vi "Auto-Calibrate.vi"(6 "Uncertainty (%) Vin":dbl=1.0, 7 "Uncertainty (%) Vout":dbl=1.0, 10 "V_in (V)":dbl=5.0) -> (0 "Uncertainty Calib Temp":dbl=1.0, 1 "Calib Temperature":dbl=292.15, 2 "Uncertainty (%) Thermistor":dbl=2.872472092283147, 3 "Calibration Resistance (ohms)":dbl=7684.457551235735)   [LabVIEW 2012]
panel:
  in  "Uncertainty (%) Resistor":dbl=1.0
  in  "Resistor (ohms)":dbl=10000.0
  in  "Uncertainty (%) Temp":dbl=1.0
  in  "Temperature (K)":dbl=292.15
  # "Options"
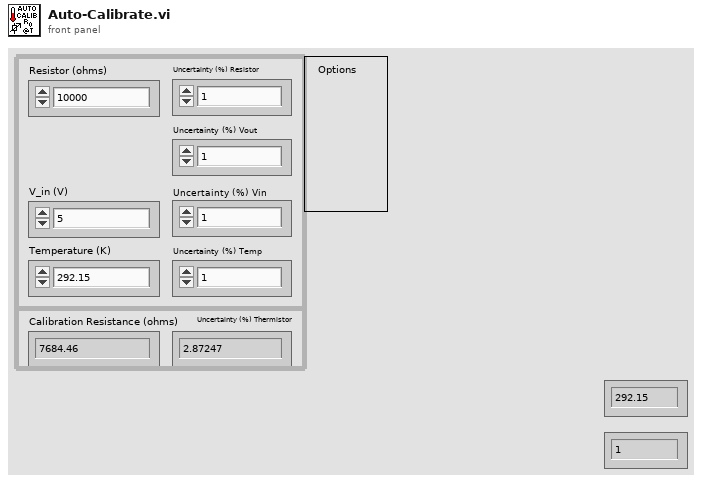
[diagram p1: front panel]
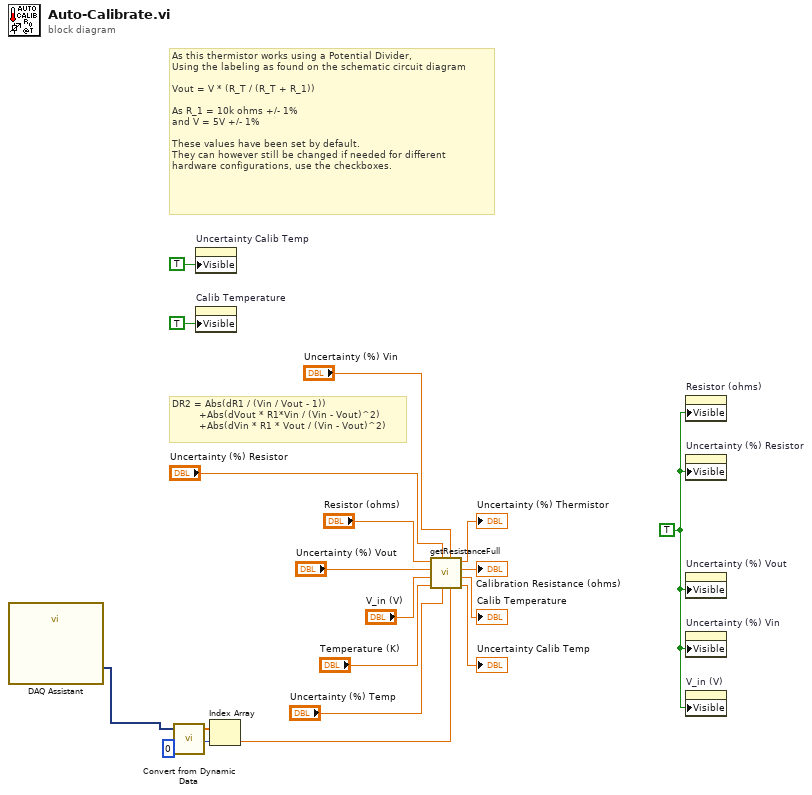
[diagram p0: block diagram]
diagram:
  w16 = TRUE ("Visible")
  # "As this thermistor works using a Potential Divider,\nUsing the labeling as found on the schematic circuit diagram\n\nVout = V * (R_T / (R_T + R_1))\n\nAs R_1 = 10k ohms +/- 1%\nand V = 5V +/- 1%\n\nThese values have been set by default.\nThey can however still be changed if needed for different \nhardware configurations, use the checkboxes."
  # "DR2 = Abs(dR1 / (Vin / Vout - 1))\n         +Abs(dVout * R1*Vin / (Vin - Vout)^2)\n         +Abs(dVin * R1 * Vout / (Vin - Vout)^2)"
  n1 = call "DAQ Assistant"() -> ("data"=w1:dynamicdata)  [unwired: 17 in, 2 out]
  n2 = call "Convert from Dynamic Data"("Dynamic Data Type"=w1) -> ("Array"=w4:dbl[])  [unwired: 3 in]
  n3 = property on="Uncertainty Calib Temp" class="DigNum (strict)"("Visible"=TRUE) -> ()  [unwired: 2 in, 2 out]
  n4 = property on="Calib Temperature" class="DigNum (strict)"("Visible"=TRUE) -> ()  [unwired: 2 in, 2 out]
  n5 = Index Array(array=w4, index=0) -> (element=w3:dbl)
  n6 = call "getResistanceFull.vi"("V_out (V)"=w3, "Uncertainty (%) Vin"="Uncertainty (%) Vin", "Uncertainty (%) Temp in"="Uncertainty (%) Temp", "Uncertainty (%) Resistor"="Uncertainty (%) Resistor", "Temperature (K) in"="Temperature (K)", "V_in (V)"="V_in (V)", "Uncertainty (%) Vout"="Uncertainty (%) Vout", "Resistor (ohms)"="Resistor (ohms)") -> ("Uncertainty (%) Temp out"=→"Uncertainty Calib Temp":dbl, "Temperature (K) out"=→"Calib Temperature":dbl, "Resistance"=→"Calibration Resistance (ohms)":dbl, "Uncertainty"=→"Uncertainty (%) Thermistor":dbl)
  n7 = property on="Resistor (ohms)" class="DigNum (strict)"("Visible"=w16) -> ()  [unwired: 2 in, 2 out]
  n8 = property on="Uncertainty (%) Resistor" class="DigNum (strict)"("Visible"=w16) -> ()  [unwired: 2 in, 2 out]
  n9 = property on="Uncertainty (%) Vout" class="DigNum (strict)"("Visible"=w16) -> ()  [unwired: 2 in, 2 out]
  n10 = property on="Uncertainty (%) Vin" class="DigNum (strict)"("Visible"=w16) -> ()  [unwired: 2 in, 2 out]
  n11 = property on="V_in (V)" class="DigNum (strict)"("Visible"=w16) -> ()  [unwired: 2 in, 2 out]
